vi "Session Json to Data Add Session - Initialize Sessions.vi"(8 "error in":errorcluster, 11 "json in":string) -> (0 "error out":errorcluster, 3 "data out":T1)   [LabVIEW 2020, in "MeasurementServerTests.lvlib"]
uses:
  MeasurementServerTests.lvlib
  Runtime/MeasurementLink Session Management/Session Reservation/Data.ctl
  Runtime/MeasurementLink Session Management/Connection Map/Connection Map.lvclass
  Runtime/MeasurementLink Session Management/IReservationObserver/IReservationObserver.lvclass
  Runtime/MeasurementLink Session Management/Session Reservation/Session and Driver Info.ctl
  Runtime/MeasurementLink Instrument/ISession Factory/ISession Factory.lvclass
  Runtime/MeasurementLink Session Management Client/RPC Messages/ni_measurementlink_sessionmanagement_v1_SessionInformation.ctl
  Runtime/MeasurementLink Session Management Client/RPC Messages/nidevice_grpc_Session.ctl
  Runtime/MeasurementLink Session Management Client/RPC Messages/ni_measurementlink_sessionmanagement_v1_ChannelMapping.ctl
  Runtime/MeasurementLink Instrument/ISession Factory/Initialize and Close Session Behavior.ctl
  Runtime/MeasurementLink Session Management Client/RPC Messages/ni_measurementlink_PinMapContext.ctl
  2dfce5ba-96f1-4d0e-9517-3e25601897e8.vi
  <vilib>/JDP Science/JSONtext/JSON text to Variant.vi
  <vilib>/JDP Science/JSONtext/LVClass Serializer/JSONtext LVClass Serializer.lvclass
  Runtime/MeasurementLink Session Management/Session Reservation/Session Reservation.lvclass
  Runtime/MeasurementLink Session Management Client/MeasurementLink Session Management Client.lvlib
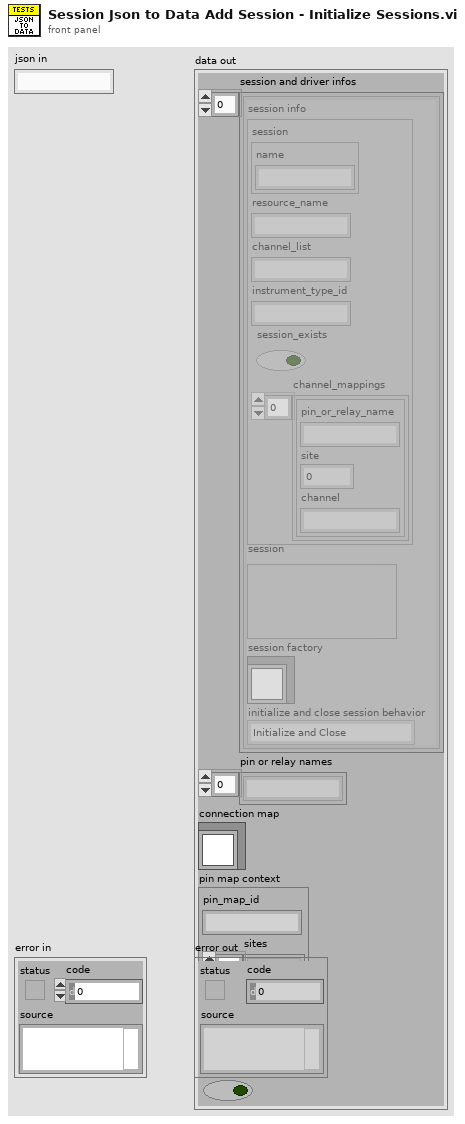
[diagram p1: front panel]
types:
  T1 = typedef "MeasurementLink Session Management.lvlib/Session Reservation.lvclass/Data.ctl" = cluster{"session and driver infos":T2[], "pin or relay names":string[], "connection map":refnum<class "Connection Map.lvclass">, "pin map context":T7, "reservation observer":refnum<class "IReservationObserver.lvclass">, "dvr valid":bool}
  T2 = typedef "MeasurementLink Session Management.lvlib/Session Reservation.lvclass/Session and Driver Info.ctl" = cluster{"session info":T3, "session":variant, "session factory":refnum<class "ISession Factory.lvclass">, "initialize and close session behavior":T6}
  T3 = typedef "MeasurementLink Session Management Client.lvlib/ni_measurementlink_sessionmanagement_v1_SessionInformation.ctl" = cluster{"session":T4, "resource_name":string, "channel_list":string, "instrument_type_id":string, "session_exists":bool, "channel_mappings":T5[]}
  T4 = typedef "MeasurementLink Session Management Client.lvlib/nidevice_grpc_Session.ctl" = cluster{"name":string}
  T5 = typedef "MeasurementLink Session Management Client.lvlib/ni_measurementlink_sessionmanagement_v1_ChannelMapping.ctl" = cluster{"pin_or_relay_name":string, "site":i32, "channel":string}
  T6 = typedef "MeasurementLink Instrument.lvlib/ISession Factory.lvclass/Initialize and Close Session Behavior.ctl" = enum16{"Initialize and Close", "Attach and Detach", "Initialize and Detach", "Attach and Close"}
  T7 = typedef "MeasurementLink Session Management Client.lvlib/ni_measurementlink_PinMapContext.ctl" = cluster{"pin_map_id":string, "sites":i32[]}
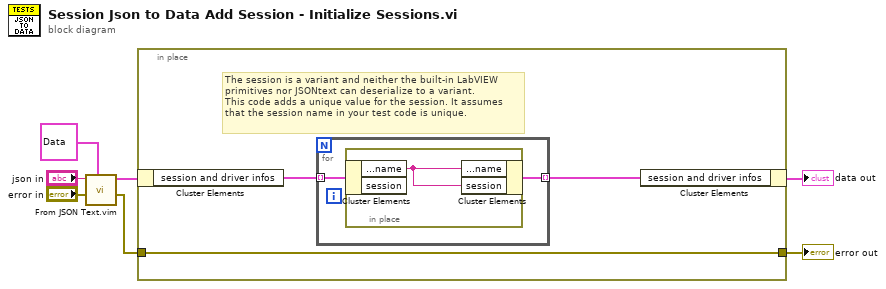
[diagram p0: block diagram]
diagram:
  n1 = call "From JSON Text.vim"("Data Type and Default Value"=T1 {"session and driver infos"=[], "pin or relay names"=[], "connection map"=refnum, "pin map context"={"pin_map_id"="", "sites"=[]}, "reservation observer"=refnum, "dvr valid"=FALSE} ("data"), "error in (no error)"="error in", "JSON"="json in") -> ("error out"=w2:errorcluster, "Data out"=w5:T1)  [unwired: 7 in]
  n2 = in-place {
    in-place-border: w2 -> [w10]
    in-place-border: [w10] -> w1
    # "The session is a variant and neither the built-in LabVIEW\nprimitives nor JSONtext can deserialize to a variant.\nThis code adds a unique value for the session. It assumes\nthat the session name in your test code is unique."
    n3 = in-place-cluster #1(w5) -> ("session and driver infos"=w9:T2[])
    n4 = for {
      tunnel: w9 -> [w12] mode=indexing
      tunnel: [w11] -> w8 mode=indexing
      n5 = in-place {
        n6 = in-place-cluster #2(w12) -> ("session info.session.name"=w13:string)  [unwired: 1 out]
        n7 = in-place-cluster #2("session info.session.name"=w13, "session"=w13) -> (w11:T2)
      }
    }
    n8 = in-place-cluster #1("session and driver infos"=w8) -> (→"data out":T1)
  }
  "error out" <- w1
